vi "test-trapezoid-profile-reaches-goal.vi"() -> (3 "Test Passed":bool)   [LabVIEW 2019]
uses:
  <vilib>/Rock Robotics/WPI/ThirdParty/JAS_Junk/TrajLib/TRAPEZOID_PROFILE_STATE.ctl
  <vilib>/Rock Robotics/WPI/ThirdParty/JAS_Junk/TrajLib/TrapProfile_ShouldFlipAcceleration.vi
  <vilib>/Rock Robotics/WPI/ThirdParty/JAS_Junk/TrajLib/TrapProfile_Direct.vi
  <vilib>/Rock Robotics/SystemInterfaces/NetworkCommunication/NetComm_UsageReport_report.vi
  <vilib>/Rock Robotics/WPI/ThirdParty/JAS_Junk/TrajLib/Util_LibraryGlobals.vi
  <vilib>/Rock Robotics/WPI/ThirdParty/JAS_Junk/TrajLib/Trajectory_Library.lvlib
panel:
  out "ApproxEquals 2":bool
  out "ApproxEquals":bool
  out "Equal":bool
  out "State":T1 {"Velocity" format="%16_6e"; "Position" format="%16_6e"}
  out "Waveform Chart":T2(graph)
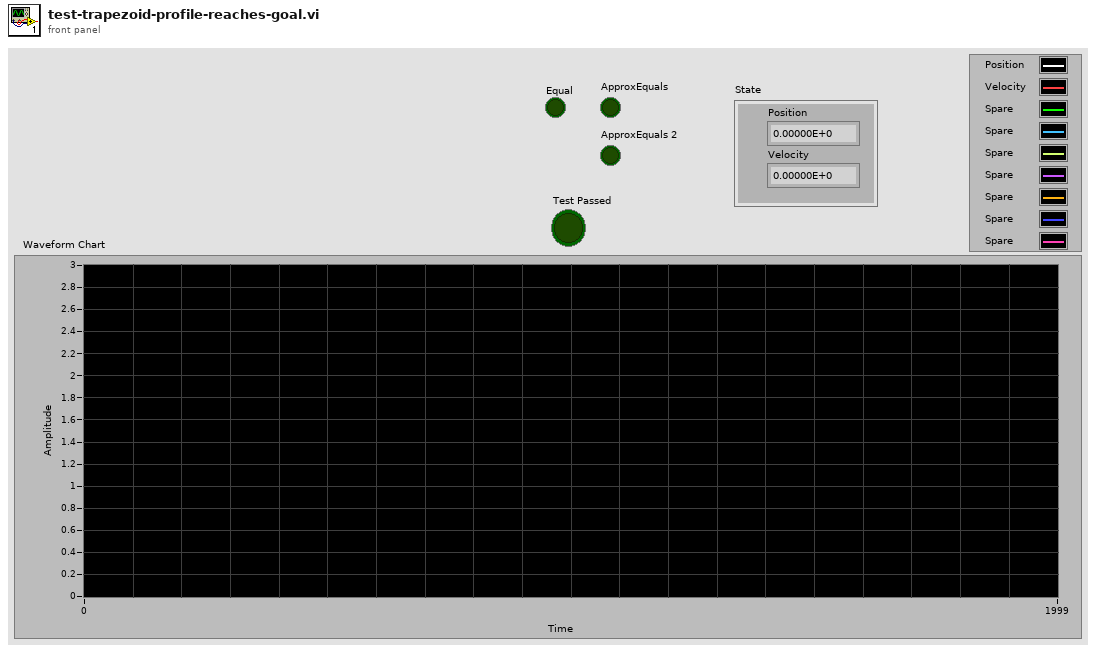
[diagram p1: front panel]
types:
  T1 = typedef "Trajectory_Library.lvlib/TRAPEZOID_PROFILE_STATE.ctl" = cluster{"Position":dbl, "Velocity":dbl}
  T2 = cluster{dbl, dbl, "Output":dbl, "Output":dbl, "Output":dbl, "Output":dbl, "Output":dbl, "Output":dbl, "Output":dbl}
  T3 = typedef "Trajectory_Library.lvlib/TRAPEZOID_PROFILE_CONSTRAINT.ctl" = cluster{"MaxVelocity":dbl, "MaxAcceleration":dbl}
  T4 = typedef "Trajectory_Library.lvlib/TRAPEZOID_PROFILE.ctl" = cluster{"EndAccel":dbl, "EndFullSpeed":dbl, "EndDecel":dbl, "Direction":i32, "Constraints":T3, "Initial":T1, "Goal":T1}
  T5 = cluster{"Position":dbl, "Velocity":dbl, "Velocity":dbl, "Velocity":dbl, "Velocity":dbl, "Velocity":dbl, "Velocity":dbl, "Velocity":dbl, "Velocity":dbl}
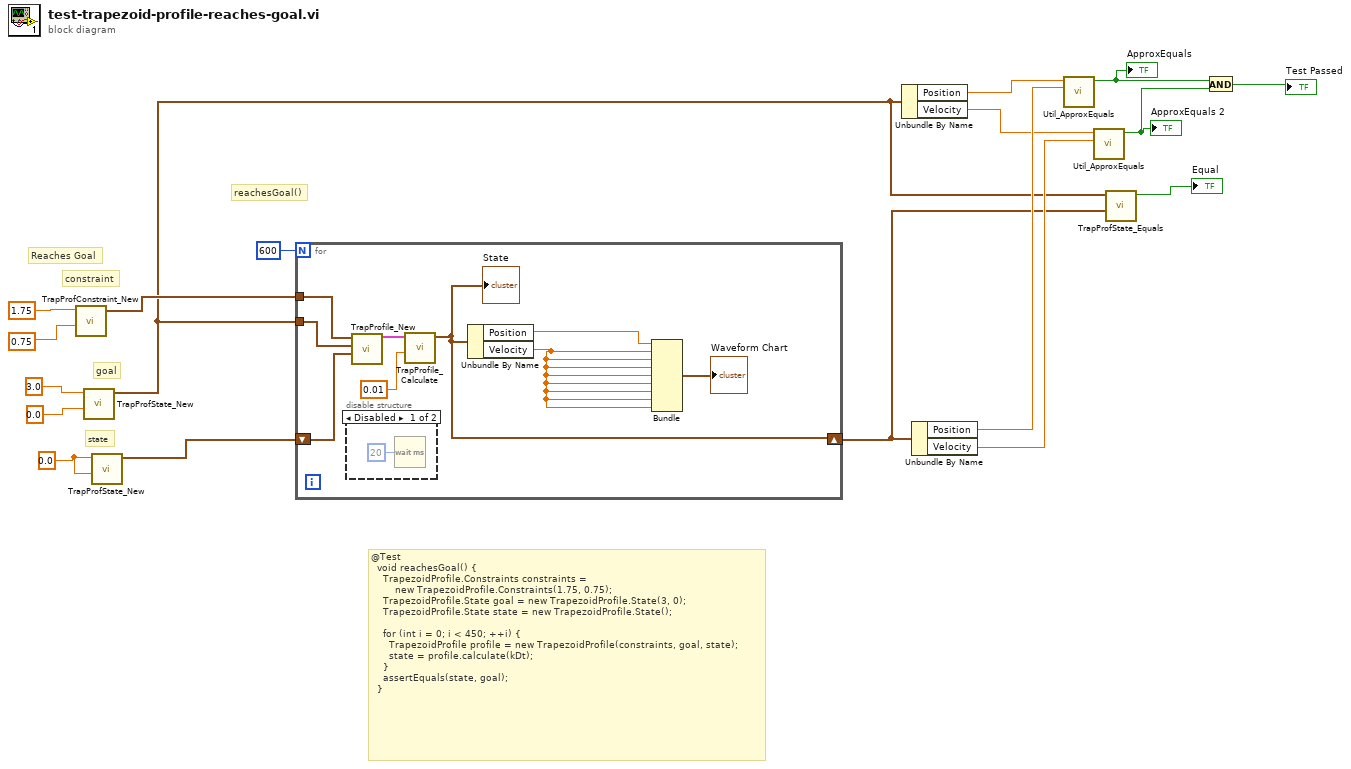
[diagram p0: block diagram]
diagram:
  w16 = 0.0 ("Position")
  # "@Test\n  void reachesGoal() {\n    TrapezoidProfile.Constraints constraints =\n        new TrapezoidProfile.Constraints(1.75, 0.75);\n    TrapezoidProfile.State goal = new TrapezoidProfile.State(3, 0);\n    TrapezoidProfile.State state = new TrapezoidProfile.State();\n\n    for (int i = 0; i < 450; ++i) {\n      TrapezoidProfile profile = new TrapezoidProfile(constraints, goal, state);\n      state = profile.calculate(kDt);\n    }\n    assertEquals(state, goal);\n  }"
  # "reachesGoal()"
  # "goal"
  # "state"
  # "Reaches Goal"
  # "constraint"
  n1 = call <vilib>:"TrapProfConstraint_New.vi"("Max Accel"=0.75, "Max Speed (M/S)"=1.75) -> ("TRAPEZOID_PROFILE_CONSTRAINT"=w12:T3)  [unwired: 9 in]
  n2 = call <vilib>:"TrapProfState_New.vi"("Velocity"=0.0, "Position"=3.0) -> ("TRAPEZOID_PROFILE_STATE"=w1:T1)  [unwired: 9 in]
  n3 = call <vilib>:"TrapProfState_New.vi"("Velocity"=w16, "Position"=w16) -> ("TRAPEZOID_PROFILE_STATE"=w11:T1)  [unwired: 9 in]
  n4 = for {
    N: 600 -> [_]
    tunnel: w12 -> [w24]
    tunnel: w1 -> [w23]
    shift-right: [w22] -> w2
    shift-left: w11 -> [w19]
    n5 = disable-structure shown="Disabled" {
      frame Disabled {
        n6 = Wait (ms)(milliseconds to wait=u32 20) -> ()  [unwired: 1 out]
      }
      frame Enabled {
      }
    }
    n7 = call <vilib>:"TrapProfile_New.vi"("Initial"=w19, "Goal"=w23, "Constraints"=w24) -> ("TRAPEZOID_PROFILE"=w21:T4)  [unwired: 8 in]
    n8 = call <vilib>:"TrapProfile_Calculate.vi"("Time"=0.01, "TRAPEZOID_PROFILE"=w21) -> ("State"=w22:T1)  [unwired: 9 in]
    "State" <- w22
    n9 = Unbundle By Name(w22) -> ("Position"=w25:dbl, "Velocity"=w26:dbl)
    n10 = Bundle("Position"=w25, "Velocity"=w26, "Velocity"=w26, "Velocity"=w26, "Velocity"=w26, "Velocity"=w26, "Velocity"=w26, "Velocity"=w26, "Velocity"=w26) -> (→"Waveform Chart":T5)  [unwired: 1 in]
  }
  n11 = Unbundle By Name(w1) -> ("Position"=w10:dbl, "Velocity"=w8:dbl)
  n12 = Unbundle By Name(w2) -> ("Position"=w9:dbl, "Velocity"=w6:dbl)
  n13 = call <vilib>:"Util_ApproxEquals.vi"("Value 2"=w9, "Value 1"=w10) -> ("ApproxEquals"=w4:bool)  [unwired: 9 in]
  "ApproxEquals" <- w4
  n14 = call <vilib>:"Util_ApproxEquals.vi"("Value 2"=w6, "Value 1"=w8) -> ("ApproxEquals"=w3:bool)  [unwired: 9 in]
  "ApproxEquals 2" <- w3
  n15 = call <vilib>:"TrapProfState_Equals.vi"("TRAPEZOID_PROFILE_STATE 2"=w2, "TRAPEZOID_PROFILE_STATE"=w1) -> ("Equal"=→"Equal":bool)  [unwired: 9 in]
  n16 = And(x=w4, y=w3) -> (x .and. y?=→"Test Passed":bool)
